vi "Status Bar.vi"(0 "Status Bar":refnum<vi>, 5 "Status":string, 11 "error in (no error)":errorcluster, 13 "Operation":T1) -> (15 "error out":errorcluster)   [LabVIEW 2014, in "Status Bar.lvlib"]
uses:
  Status Bar.lvlib
  Typedefs/Status Bar Operation.ctl
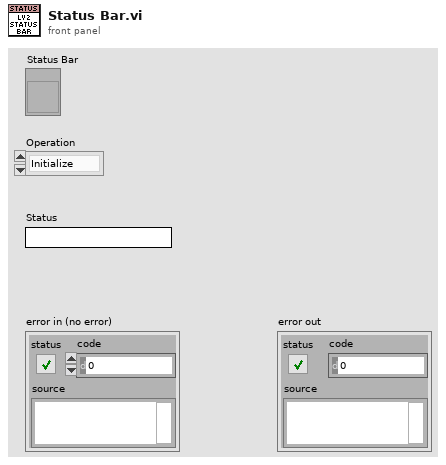
[diagram p1: front panel]
types:
  T1 = typedef "Status Bar.lvlib/Status Bar Operation.ctl" = enum16{"Initialize", "Update", "Clear", "Close"}
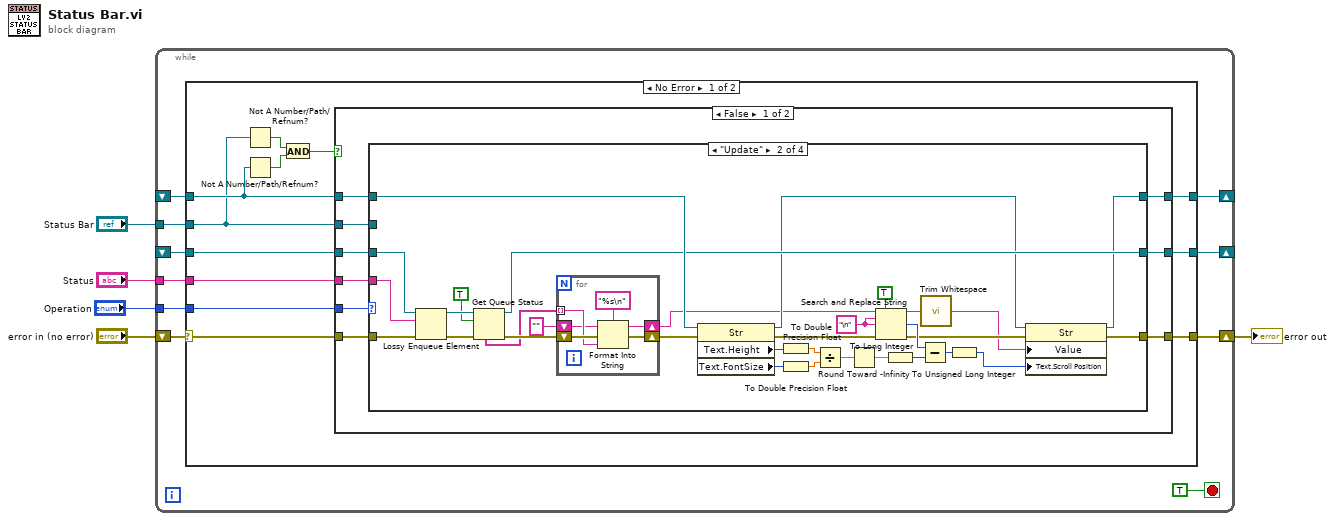
[diagram p0: block diagram]
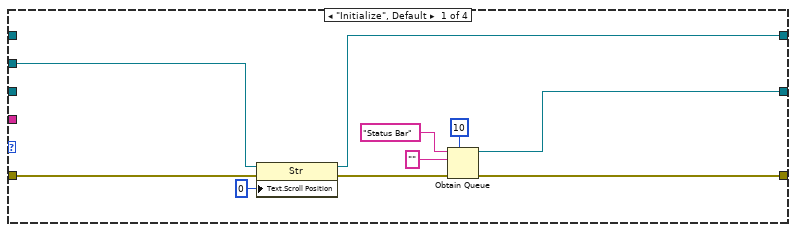
[diagram p2: hidden frame]
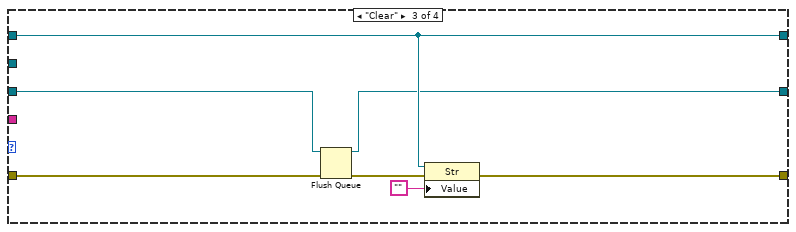
[diagram p3: hidden frame]
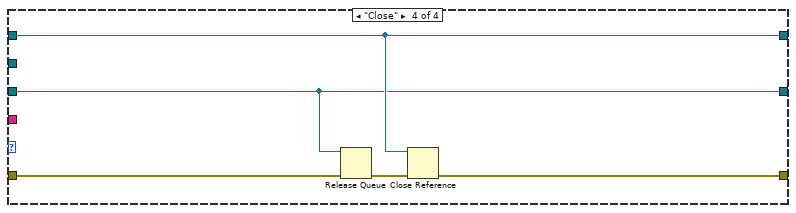
[diagram p4: hidden frame]
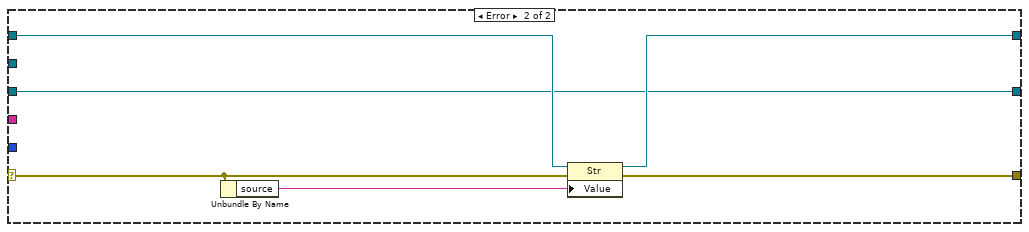
[diagram p6: hidden frame]
diagram:
  n1 = while {
    shift-right: [w14] -> _
    shift-left: _ -> [w15]
    tunnel: "Operation" -> [w13]
    tunnel: "Status Bar" -> [w12]
    shift-right: [w10] -> w3
    shift-left: "error in (no error)" -> [w11]
    tunnel: "Status" -> [w8]
    shift-right: [w7] -> _
    shift-left: _ -> [w6]
    stop <- TRUE stop-if-true
    n2 = case shown="No Error" w11 {
      selector: w11 -> [w25 w102]
      tunnel: w15 -> [w17 w104]
      tunnel: [w27 w103] -> w14
      tunnel: w13 -> [w26 _]
      tunnel: w12 -> [w16 _]
      tunnel: [w24 w105] -> w10
      tunnel: w8 -> [w23 _]
      tunnel: [w22 w100] -> w7
      tunnel: w6 -> [w21 w100]
      frame No Error {
        n3 = Not A Number/Path/Refnum?(number/path/refnum=w16) -> (NaN/Path/Refnum?=w20:bool)
        n4 = Not A Number/Path/Refnum?(number/path/refnum=w17) -> (NaN/Path/Refnum?=w19:bool)
        n5 = And(x=w20, y=w19) -> (x .and. y?=w18:bool)
        n6 = case shown="False" w18 {
          tunnel: w17 -> [w36 w99]
          tunnel: [w35 w99] -> w27
          tunnel: w26 -> [w34 _]
          tunnel: w16 -> [w33 _]
          tunnel: w25 -> [w32 w97]
          tunnel: [w31 w97] -> w24
          tunnel: w23 -> [w30 _]
          tunnel: [w29 w98] -> w22
          tunnel: w21 -> [w28 w98]
          frame False {
            n7 = case shown="\"Update\"" w34 {
              tunnel: w36 -> [_ w75 w89 w95]
              tunnel: [w38 w52 w89 w95] -> w35
              tunnel: w33 -> [w39 _ _ _]
              tunnel: w32 -> [w41 w77 w90 w94]
              tunnel: [w46 w78 w91 w96] -> w31
              tunnel: w30 -> [_ w76 _ _]
              tunnel: [w43 w73 w87 w92] -> w29
              tunnel: w28 -> [_ w74 w88 w92]
              frame "Initialize", Default {
                n8 = property class="Str"(reference=w39, error in=w41, "Text.Scroll Position"=u32 0) -> (reference out=w38:refnum<vi>, error out=w40:errorcluster)
                n9 = Obtain Queue(max queue size (-1, unlimited)=10, name (unnamed)="Status Bar", element data type="" ("Status"), error in (no error)=w40) -> (queue out=w43:refnum<queue>, error out=w46:errorcluster)  [unwired: 1 in, 1 out]
              }
              frame "Update" {
                w58 = "\n" ("String")
                n10 = Lossy Enqueue Element(queue=w74, element=w76, error in (no error)=w77) -> (queue out=w70:refnum<queue>, error out=w72:errorcluster)  [unwired: 2 out]
                n11 = Get Queue Status(queue=w70, return elements? (F)=TRUE, error in (no error)=w72) -> (queue out=w73:refnum<queue>, error out=w71:errorcluster, elements=w68:string[])  [unwired: 5 out]
                n12 = for {
                  shift-right: [w84] -> w66
                  shift-left: w71 -> [w81]
                  tunnel: w68 -> [w80] mode=indexing
                  shift-right: [w82] -> w48
                  shift-left: "" ("Status") -> [w79]
                  n13 = Format Into String(format string="%s\n" ("Status"), initial string=w79, error in=w81, w80) -> (resulting string=w82:string, error out=w84:errorcluster)
                }
                n14 = property class="Str"(reference=w75, error in=w66) -> (reference out=w63:refnum<vi>, error out=w57:errorcluster, "Text.Height"=w65:u32, "Text.FontSize"=w64:u32)
                n15 = To Double Precision Float(number=w65) -> (double precision float=w54:dbl)
                n16 = To Double Precision Float(number=w64) -> (double precision float=w55:dbl)
                n17 = Divide(x=w54, y=w55) -> (x/y=w49:dbl)
                n18 = Round Toward -Infinity(1:w49) -> (0:w47:dbl)
                n19 = Search and Replace String(replace all?=TRUE ("replace all? (F)"), input string=w48, search string=w58, replace string=w58, error in=w57) -> (result string=w51:string, number of replacements=w60:i32, error out=w56:errorcluster)  [unwired: 3 in, 1 out]
                n20 = To Long Integer(number=w47) -> (32bit integer=w61:i32)
                n21 = Subtract(x=w60, y=w61) -> (x-y=w62:i32)
                n22 = call <vilib>:"Trim Whitespace.vi"("string"=w51) -> ("trimmed string"=w50:string)  [unwired: 1 in]
                n23 = To Unsigned Long Integer(number=w62) -> (unsigned 32bit integer=w53:u32)
                n24 = property class="Str"(reference=w63, error in=w56, "Value"=w50, "Text.Scroll Position"=w53) -> (reference out=w52:refnum<vi>, error out=w78:errorcluster)
              }
              frame "Clear" {
                n25 = Flush Queue(queue=w88, error in (no error)=w90) -> (queue out=w87:refnum<queue>, error out=w85:errorcluster)  [unwired: 1 out]
                n26 = property class="Str"(reference=w89, error in=w85, "Value"="") -> (error out=w91:errorcluster)  [unwired: 1 out]
              }
              frame "Close" {
                n27 = Release Queue(queue=w92, error in (no error)=w94) -> (error out=w93:errorcluster)  [unwired: 1 in, 2 out]
                n28 = Close Reference(reference=w95, error in (no error)=w93) -> (error out=w96:errorcluster)
              }
            }
          }
          frame True {
          }
        }
      }
      frame Error {
        n29 = Unbundle By Name(w102) -> ("source"=w101:string)
        n30 = property class="Str"(reference=w104, error in=w102, "Value"=w101) -> (reference out=w103:refnum<vi>, error out=w105:errorcluster)
      }
    }
  }
  "error out" <- w3
